vi "Read 1 Register.vi"(8 "Error In":errorcluster, 10 "Register Address":u8, 11 "Adept Config":T1) -> (0 "Error Out":errorcluster, 2 "Data":u8, 3 "Adept Config":T1)   [LabVIEW 2011, in "LVH-Adept.lvlib"]
uses:
  <vilib>/LabVIEW Hacker/Adept/LVH-Adept.lvlib
  <vilib>/LabVIEW Hacker/Adept/Private/Type Defs/Device Config.ctl
  <vilib>/LabVIEW Hacker/Adept/Private/Type Defs/Status.ctl
  <vilib>/LabVIEW Hacker/Adept/Private/DEPP/DEPP.lvlib
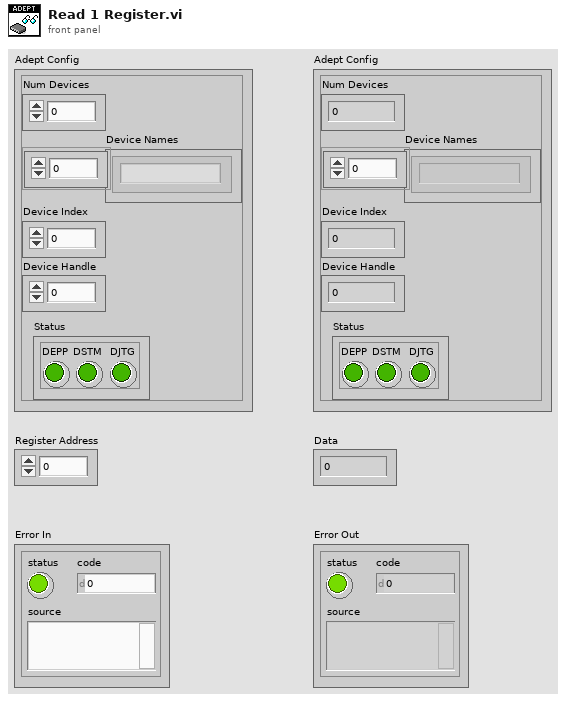
[diagram p1: front panel]
types:
  T1 = typedef "LVH-Adept.lvlib/Device Config.ctl" = cluster{"Num Devices":i32, "Device Names":string[], "Device Index":u16, "Device Handle":u32, "Status":T2}
  T2 = typedef "LVH-Adept.lvlib/Status.ctl" = cluster{"DEPP":bool, "DSTM":bool, "DJTG":bool}
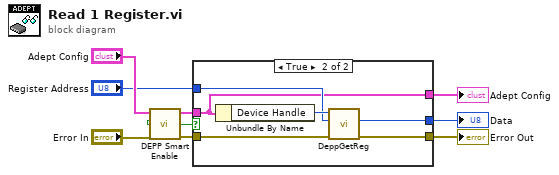
[diagram p0: block diagram]
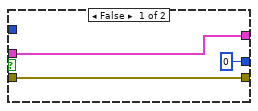
[diagram p2: hidden frame]
diagram:
  n1 = call <vilib>:"DEPP Smart Enable.vi"("Error In"="Error In", "Adept Config"="Adept Config") -> ("Error Out"=w7:errorcluster, "Success?"=w6:bool, "Adept Config"=w2:T1)  [unwired: 7 in]
  n2 = case shown="True" w6 {
    tunnel: w7 -> [w12 w18]
    tunnel: w2 -> [w11 w13]
    tunnel: "Register Address" -> [_ w16]
    tunnel: [w12 w15] -> w4
    tunnel: [u8 0 ("Data") w14] -> w3
    tunnel: [w11 w13] -> w1
    frame False {
    }
    frame True {
      n3 = Unbundle By Name(w13) -> ("Device Handle"=w17:u32)
      n4 = call <vilib>:"DeppGetReg.vi"("Error In"=w18, "Address"=w16, "Device Handle"=w17) -> ("Error Out"=w15:errorcluster, "Data"=w14:u8)  [unwired: 6 in, 1 out]
    }
  }
  "Data" <- w3
  "Error Out" <- w4
  "Adept Config" <- w1
